vi "Kundendaten.vi"(8 "error in (no error)":errorcluster) -> (0 "error out":errorcluster)   [LabVIEW 2023]
uses:
  <vilib>/Utility/miscctls.llb/LVRectTypeDef.ctl
panel:
  in  "Firmename":string
  in  "PLZ":dbl
  in  "Ort":string
  in  "Straße":string
  out "Firma":bool
  in  "Reserve Schalter 3":bool
  in  "Reserve Schalter 2":bool
  in  "Reserve Schalter":bool
  in  "Stop Button":bool
  in  "Nachname":string
  in  "Vorname":string
  in  "Daten speichern":bool
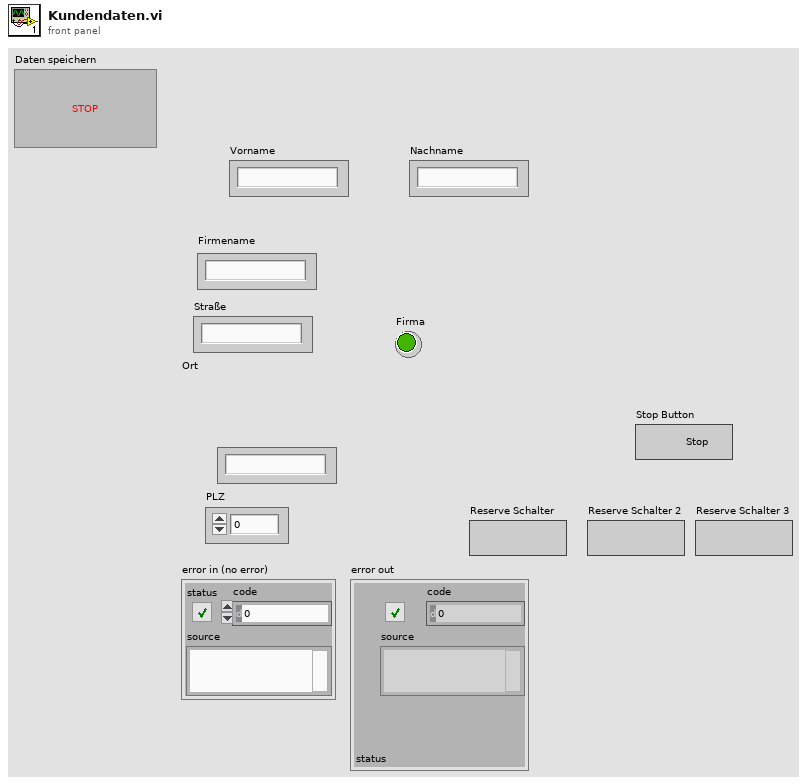
[diagram p1: front panel]
types:
  T1 = typedef "LVRectTypeDef.ctl" = cluster{"Left":i16, "Top":i16, "Right":i16, "Bottom":i16}
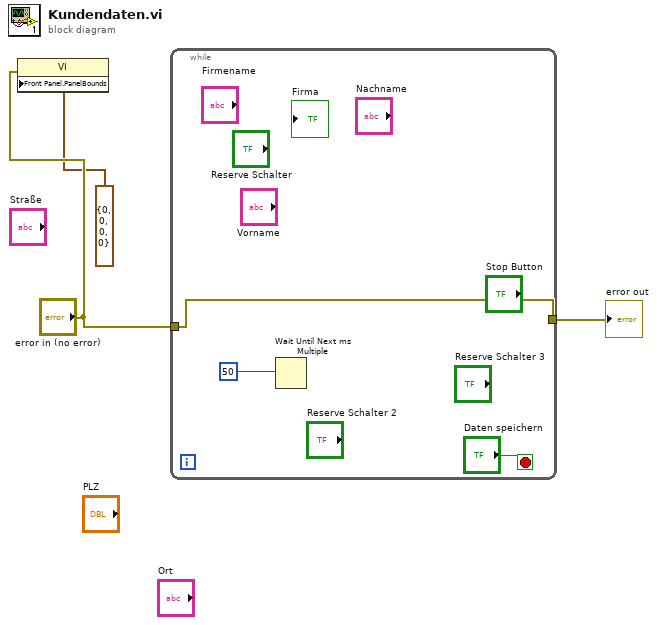
[diagram p0: block diagram]
diagram:
  n1 = property class="VI"(error in="error in (no error)", "Front Panel.PanelBounds"=T1 {"Left"=0, "Top"=0, "Right"=0, "Bottom"=0} ("Front Panel Window:Panel Bounds")) -> ()  [unwired: 1 in, 2 out]
  n2 = while {
    tunnel: "error in (no error)" -> [w5]
    tunnel: [w5] -> w2
    stop <- "Daten speichern" stop-if-true
    n3 = Wait Until Next ms Multiple(millisecond multiple=u32 50 ("millisecond timer value")) -> ()  [unwired: 1 out]
  }
  "error out" <- w2
